vi "VI Server_Get Text Ring Item Names_SpreadSheetStr.vi"(7 "Label":string, 8 "error in":errorcluster, 9 "Single Instance (T)":bool=TRUE, 11 "VI Server Cluster":T1) -> (0 "error out":errorcluster, 1 "Control Reference":refnum<vi>, 2 "Strings [].Spreadsheet STR":string, 3 "VI Server Custer.DUP":T1={"Labels"=["Label", "Size", "Font", "Heght", "Width", "Ledding Denominator", "Ledding Nominator", "Label Number", "Microstep Resolution", "X", "Y", "Z", "Italic?", "Underlined?"], "Refs"=[], "VI Ref"=refnum}, 4 "Value":u16, 6 "Label.Text DUP":string)   [LabVIEW 2020, in "VI Server Toolkit LV2013.lvlib"]
doc: "Returns item names (STR array) of the Text Ring converted into a spreadsheet string.\n\nUsed for saving the text ring contents into configuration file."
uses:
  VI Server Toolkit LV2013.lvlib
  VI Server_TypeDefs/VI Server_RefsCluster.ctl
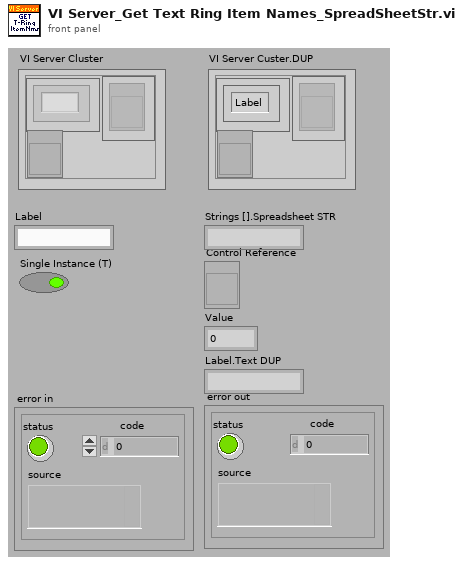
[diagram p1: front panel]
types:
  T1 = typedef "VI Server_RefsCluster.ctl" = cluster{"Labels":string[], "Refs":refnum<vi>[], "VI Ref":refnum<vi>}
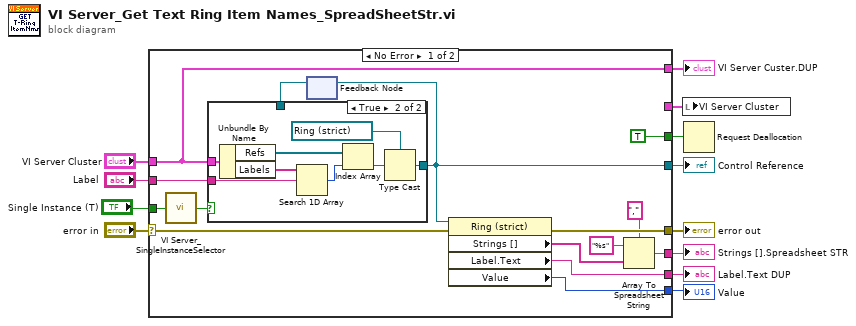
[diagram p0: block diagram]
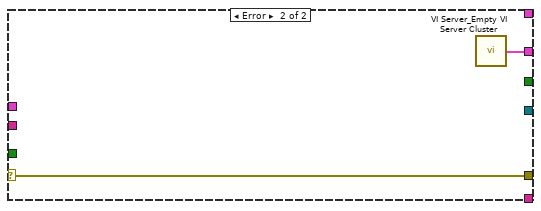
[diagram p3: hidden frame]
diagram:
  n1 = case shown="No Error" "error in" {
    selector: "error in" -> [w26 w38]
    tunnel: "Label" -> [w27 _]
    tunnel: "VI Server Cluster" -> [w23 _]
    tunnel: [w25 w38] -> w12
    tunnel: [w14 _] -> w8
    tunnel: [w24 _] -> w7
    tunnel: [w23 _] -> w6
    tunnel: [w22 _] -> w5
    tunnel: [w18 _] -> w4
    tunnel: [TRUE _] -> w3
    tunnel: [_ w37] -> w2
    tunnel: "Single Instance (T)" -> [w15 _]
    frame No Error {
      n2 = call "VI Server_SingleInstanceSelector.vi"("Single Instance (T)"=w15) -> ("Single Instance.OUT"=w16:bool)  [unwired: 6 in]
      n3 = feedback #1() -> (w13:refnum<vi>)  [unwired: 1 in]
      n4 = case shown="True" w16 {
        tunnel: w27 -> [_ w35]
        tunnel: [w28 w30] -> w14
        tunnel: w23 -> [_ w29]
        tunnel: w13 -> [w28 _]
        frame False {
        }
        frame True {
          n5 = Unbundle By Name(w29) -> ("Refs"=w33:refnum<vi>[], "Labels"=w36:string[])
          n6 = Search 1D Array(1D array=w36, element=w35) -> (index of element=w34:i32)  [unwired: 1 out]
          n7 = Index Array(array=w33, index=w34) -> (element=w32:refnum<vi>)
          n8 = Type Cast(type=refnum<vi> refnum ("Ring"), x=w32) -> (*(type *) &x=w30:refnum<vi>)
        }
      }
      n9 = feedback-in #1(w14) -> ()
      n10 = property class="Ring (strict)"(reference=w14, error in=w26) -> (error out=w25:errorcluster, "Strings []"=w21:string[], "Label.Text"=w24:string, "Value"=w22:u16)  [unwired: 1 out]
      n11 = Array To Spreadsheet String(delimiter (Tab)=",", array=w21, 3:"%s" ("format string")) -> (spreadsheet string=w18:string)
    }
    frame Error {
      n12 = call "VI Server_Empty VI Server Cluster.vi"() -> ("VI Server Cluster"=w37:T1)  [unwired: 7 in]
    }
  }
  "error out" <- w12
  "VI Server Custer.DUP" <- w6
  "Control Reference" <- w8
  "Label.Text DUP" <- w7
  "Value" <- w5
  "Strings [].Spreadsheet STR" <- w4
  n13 = local write "VI Server Cluster"(w2) -> ()
  n14 = Request Deallocation(w3) -> ()
